vi "TermistorTemp.vi"(0 "AI0-PORT":tag, 5 "stop":bool) -> (14 "Temperatur fra termistor":dbl, 19 "Thermistor Modstand":dbl)   [LabVIEW 2022 SP3]
doc: "* Temperaturmåling fra NTC Termistor *\nDenne SubVi anvender AI0+ porten til at måle spændingen i knudepunktet på spændingsdeleren.\nDette opsæt består af:\n- 1. stk 10K-Ohm modstand.\n- 1. stk NTC-Termistor.\n\nOutput kanaler på MyDAQ til målinger:\n- 5V.\n\nInput kanaler på MyDAQ til målinger:\n- AI0 +\n- AI0 -\n- AGND (& evt. GND ** Better Safe then sorry **)\n\nEt eksempel på data output:\nVolt ud: 2.467501 \n\nHerfra er spændingsdeler formlen opsat så volt ud kan omdannes til modstanden over termistoren gennem følgende formel:\n- R_2 = R_1 * (V_out / (V_in - V_out))\n\nDen fundne modstand omsættes herefter til en temperatur gennem Steinhart-Hart ligningen:\n1/(A0 + A1 * (ln(R_2)) + A2 * (ln(R_2)^2) + A3 * (ln(R_2)^3))"
uses:
  <vilib>/Utility/error.llb/DialogType.ctl
  <vilib>/DAQmx/read.llb/DAQmx Read (Analog DBL 1Chan 1Samp).vi
  <vilib>/DAQmx/create/channels.llb/DAQmx Create Channel (AI-Voltage-Basic).vi
  <vilib>/DAQmx/miscellaneous.llb/DAQmx Fill In Error Info.vi
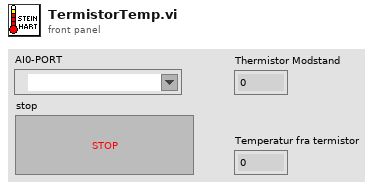
[diagram p1: front panel]
types:
  T1 = typedef "DialogType.ctl" = u16
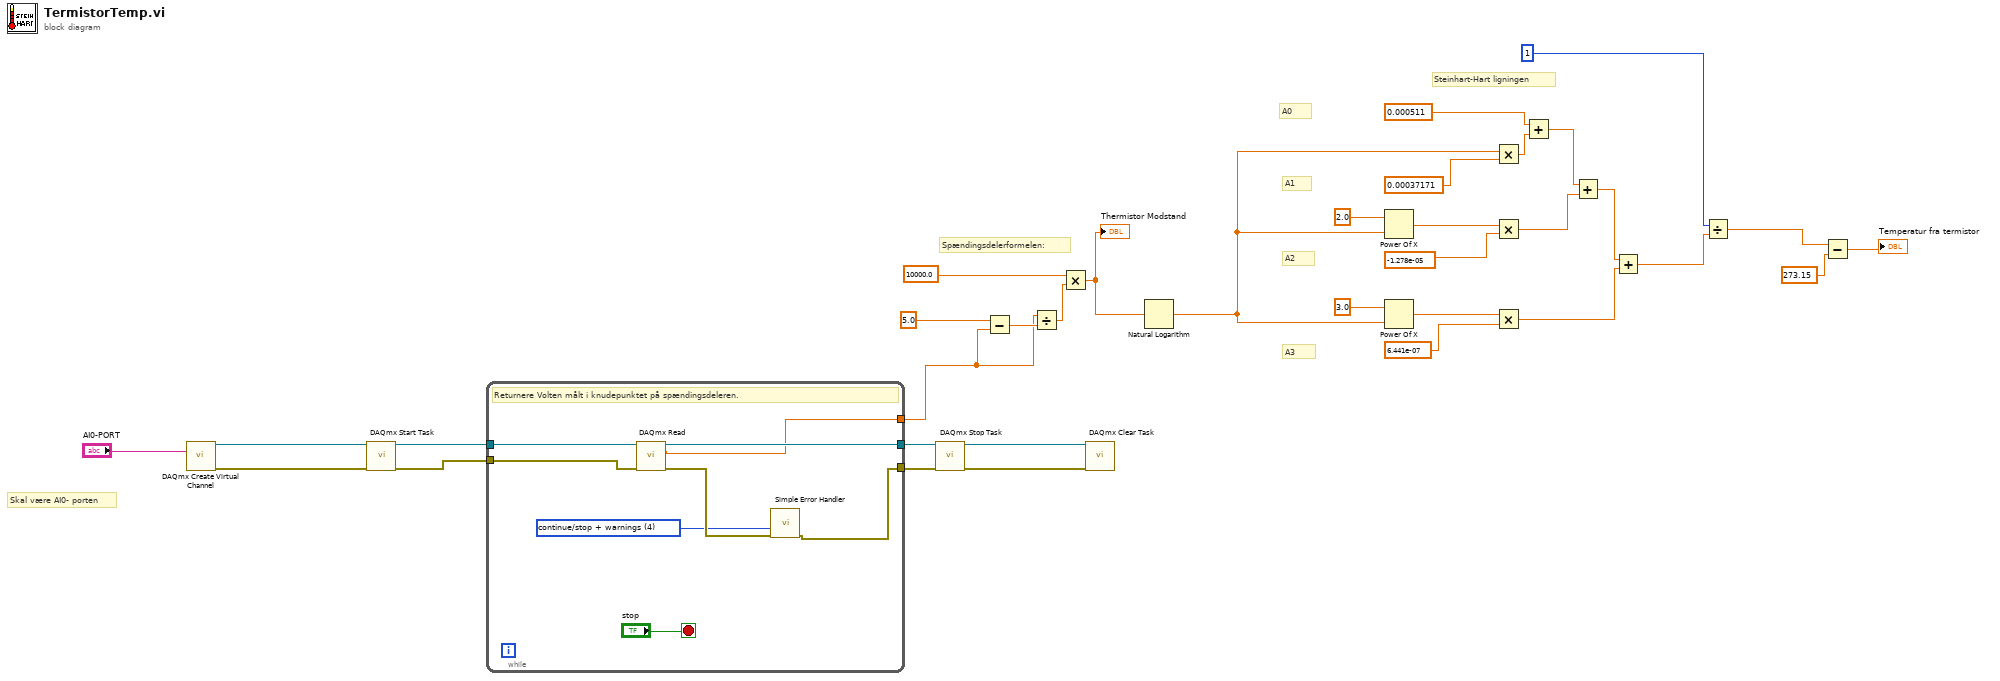
[diagram p0: block diagram]
diagram:
  # "Steinhart-Hart ligningen"
  # "A3"
  # "A2"
  # "A1"
  # "A0"
  # "Spændingsdelerformelen:"
  # "Skal være AI0- porten"
  n1 = call-poly <vilib>:"DAQmx Create Virtual Channel.vi"("physical channels"="AI0-PORT") -> ("task out"=w33:refnum<k21>, "error out"=w32:errorcluster)  [unwired: 13 in]
  n2 = call <vilib>:"DAQmx Start Task.vi"("task/channels in"=w33, "error in"=w32) -> ("task out"=w31:refnum<k21>, "error out"=w30:errorcluster)  [unwired: 12 in]
  n3 = while {
    tunnel: w31 -> [w42]
    tunnel: w30 -> [w41]
    tunnel: [w38] -> w27
    tunnel: [w37] -> w26
    tunnel: [w36] -> w21
    stop <- "stop" stop-if-true
    w39 = T1 4 items=["no dialog", "OK message", "continue or stop message", "OK message + warnings", "continue/stop + warnings"] ("type of dialog (OK msg:1)")
    # "Returnere Volten målt i knudepunktet på spændingsdeleren."
    n4 = call-poly <vilib>:"DAQmx Read.vi"("task/channels in"=w42, "error in"=w41) -> ("task out"=w38:refnum<k21>, "data"=w36:dbl, "error out"=w40:errorcluster)  [unwired: 11 in]
    n5 = call <vilib>:"Simple Error Handler.vi"("type of dialog (OK msg:1)"=w39, "error in (no error)"=w40) -> ("error out"=w37:errorcluster)  [unwired: 3 in, 4 out]
  }
  n6 = call <vilib>:"DAQmx Stop Task.vi"("task/channels in"=w27, "error in"=w26) -> ("task out"=w29:refnum<k21>, "error out"=w28:errorcluster)  [unwired: 12 in]
  n7 = Subtract(x=5.0, y=w21) -> (x-y=w25:dbl)
  n8 = Divide(x=w21, y=w25) -> (x/y=w24:dbl)
  n9 = Multiply(x=10000.0, y=w24) -> (x*y=w19:dbl)
  "Thermistor Modstand" <- w19
  n10 = call <vilib>:"DAQmx Clear Task.vi"("task in"=w29, "error in"=w28) -> ()  [unwired: 13 in, 1 out]
  n11 = Natural Logarithm(1:w19) -> (0:w8:dbl)
  n12 = Power Of X(1:w8, 2:2.0 ("y")) -> (0:w12:dbl)
  n13 = Power Of X(1:w8, 2:3.0 ("y")) -> (0:w7:dbl)
  n14 = Multiply(x=w8, y=0.00037171) -> (x*y=w15:dbl)
  n15 = Multiply(x=w12, y=-1.278e-05) -> (x*y=w10:dbl)
  n16 = Multiply(x=w7, y=6.441e-07) -> (x*y=w5:dbl)
  n17 = Add(x=0.000511, y=w15) -> (x+y=w14:dbl)
  n18 = Add(x=w14, y=w10) -> (x+y=w4:dbl)
  n19 = Add(x=w4, y=w5) -> (x+y=w18:dbl)
  n20 = Divide(x=1, y=w18) -> (x/y=w2:dbl)
  n21 = Subtract(x=w2, y=273.15) -> (x-y=→"Temperatur fra termistor":dbl)
